vi "ConfigFunc.vi"(6 "isRampable? (True":bool=TRUE, 7 "Num Layouts (ignored)":i32, 8 "error in (no error)":errorcluster, 9 "isVariable? (True)":bool=TRUE, 10 "Disableable? (True)":bool=TRUE, 11 "Column in":refnum<class "Column.lvclass">) -> (0 "error out":errorcluster, 3 "Column out":refnum<class "Column.lvclass">)   [LabVIEW 2013, in "Column.lvclass"]
doc: "Initialize functionality booleans (which are never changed).\nIf \"Disableable?\" is set true (false) then certain master modes can(not) prevent the user from changing it's value on a given line. If a column \"isVariable?\" it presents right-click menu items for variables. Both of these are typically TRUE for slave devices.\n\nAlso initialize the approprite \"Num Layouts\" if passed number > 0. For Num Layouts < 1, just pass through whatever layouts exist."
uses:
  Column.lvclass
  Column.lvclass/Column.ctl
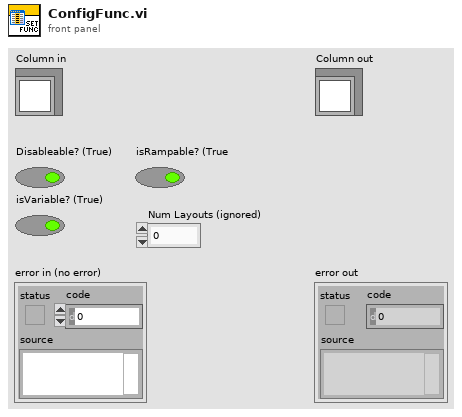
[diagram p1: front panel]
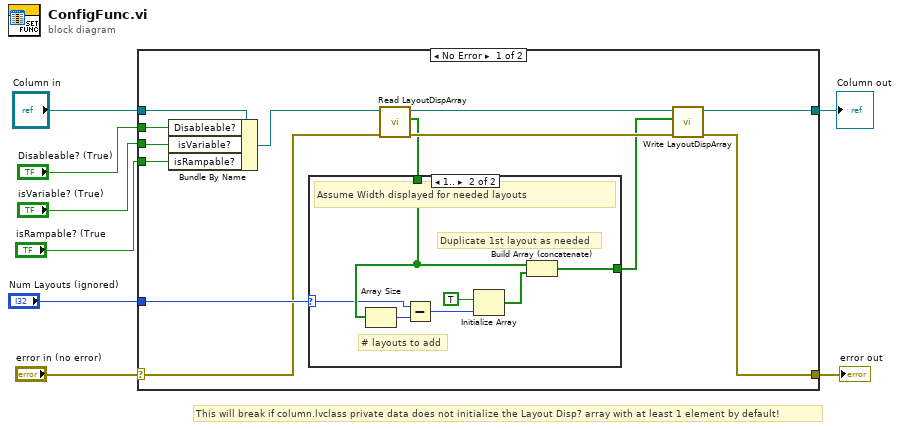
[diagram p0: block diagram]
diagram:
  # "This will break if column.lvclass private data does not initialize the Layout Disp? array with at least 1 element by default!"
  n1 = case shown="No Error" "error in (no error)" {
    selector: "error in (no error)" -> [w14 w31]
    tunnel: [w20 w31] -> w7
    tunnel: [w21 w30] -> w5
    tunnel: "Column in" -> [w13 w30]
    tunnel: "Disableable? (True)" -> [w11 _]
    tunnel: "isVariable? (True)" -> [w10 _]
    tunnel: "Num Layouts (ignored)" -> [w16 _]
    tunnel: "isRampable? (True" -> [w9 _]
    frame No Error {
      n2 = Bundle By Name(cluster=w13, "Disableable?"=w11, "isVariable?"=w10, "isRampable?"=w9) -> (w12:refnum<class "Column.lvclass">)
      n3 = call "Read LayoutDispArray.vi"("error in (no error)"=w14, "Column in"=w12) -> ("error out"=w18:errorcluster, "Layout disp? array"=w17:bool[], "Column out"=w19:refnum<class "Column.lvclass">)  [unwired: 7 in]
      n4 = case shown="1.." w16 {
        selector: w16 -> [_ w23]
        tunnel: w17 -> [w22 w24]
        tunnel: [w22 w27] -> w15
        frame Default {
          # "Don't modify layouts if passed \"Num Layouts\" < 1!"
        }
        frame 1.. {
          # "Duplicate 1st layout as needed"
          # "# layouts to add"
          # "Assume Width displayed for needed layouts"
          n5 = Array Size(array=w24) -> (size(s)=w29:i32)
          n6 = Subtract(x=w23, y=w29) -> (x-y=w28:i32)
          n7 = Initialize Array(TRUE, w28) -> (w25:bool[])
          n8 = Build Array (concatenate)(w24, w25) -> (w27:bool[])
        }
      }
      n9 = call "Write LayoutDispArray.vi"("error in (no error)"=w18, "Layout disp? array"=w15, "Column in"=w19) -> ("error out"=w20:errorcluster, "Column out"=w21:refnum<class "Column.lvclass">)  [unwired: 7 in]
    }
    frame Error {
    }
  }
  "error out" <- w7
  "Column out" <- w5
